vi "DynamicCursor.vi"() -> ()   [LabVIEW 2013]
doc: "This VI show how to create dynamic cursor."
uses:
  <vilib>/Utility/miscctls.llb/LVPointDoubleTypeDef.ctl
  <vilib>/Utility/miscctls.llb/LVCursorListTypeDef.ctl
panel:
  in  "Active Cursor":u32=3
  in  "Cursor.Cursor Position":T1
  out "XY Graph":cluster{"X":dbl, "Y":dbl}[](graph)
  # "1 Run this VI\n2 Change Cursor position\n3 Change Active Cursor"
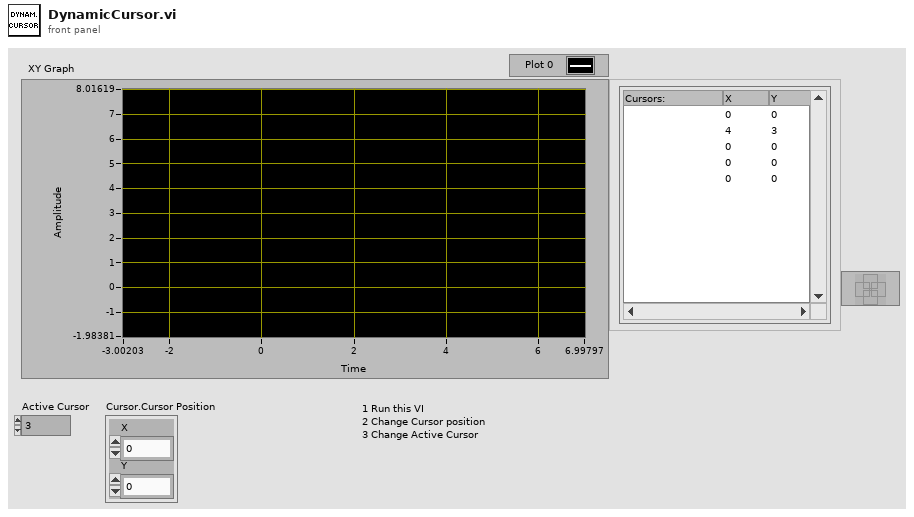
[diagram p1: front panel]
types:
  T1 = typedef "LVPointDoubleTypeDef.ctl" = cluster{"X":dbl, "Y":dbl}
  T2 = typedef "LVCursorListTypeDef.ctl" = cluster{"Name":string, "Color":u32, "Style":u8, "Point Style":u8, "Name Visible":bool, "Allow Drag":bool, "Cursor Mode":u32, "Plot":i32, "Index":i32, "Position":cluster{"X":dbl, "Y":dbl}, "X Scale":u32, "Y Scale":u32, "Watch Plots":i32[], "Watch All Plots":bool, "Plot Area":i32, "Label Offset":cluster{"X":dbl, "Y":dbl}}[]
  T3 = cluster{"Name":string, "Color":u32, "Style":u8, "Point Style":u8, "Name Visible":bool, "Allow Drag":bool, "Cursor Mode":u32, "Plot":i32, "Index":i32, "Position":cluster{"X":dbl, "Y":dbl}, "X Scale":u32, "Y Scale":u32, "Watch Plots":i32[], "Watch All Plots":bool, "Plot Area":i32, "Label Offset":cluster{"X":dbl, "Y":dbl}}
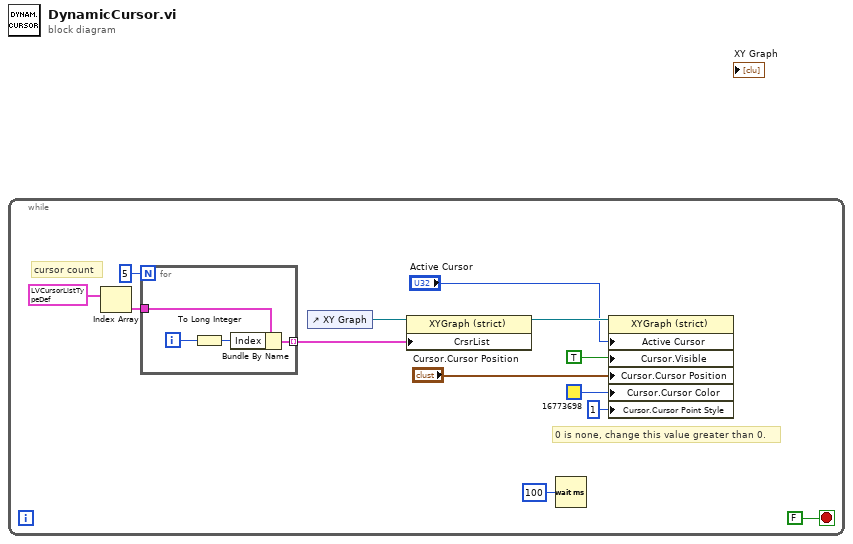
[diagram p0: block diagram]
diagram:
  n1 = while {
    stop <- FALSE stop-if-true
    # "cursor count"
    # "0 is none, change this value greater than 0."
    n2 = Index Array(array=T2 [{"Name"="", "Color"=0, "Style"=0, "Point Style"=0, "Name Visible"=FALSE, "Allow Drag"=FALSE, "Cursor Mode"=0, "Plot"=0, "Index"=0, "Position"={"X"=0.0, "Y"=0.0}, "X Scale"=0, "Y Scale"=0, "Watch Plots"=[], "Watch All Plots"=FALSE, "Plot Area"=0, "Label Offset"={"X"=0.0, "Y"=0.0}}] ("Cursor List")) -> (element=w7:T3)  [unwired: 1 in]
    n3 = for {
      N: 5 -> [_]
      tunnel: w7 -> [w17]
      tunnel: [w15] -> w6 mode=indexing
      i -> [w16]
      n4 = To Long Integer(number=w16) -> (32bit integer=w14:i32)
      n5 = Bundle By Name(cluster=w17, "Index"=w14) -> (w15:T3)
    }
    n6 = control-ref of="XY Graph"() -> (w11:refnum<vi>)
    n7 = property class="XYGraph (strict)"(reference=w11, "CrsrList"=w6) -> (reference out=w10:refnum<vi>)  [unwired: 1 in, 1 out]
    n8 = Wait (ms)(milliseconds to wait=u32 100) -> ()  [unwired: 1 out]
    n9 = property class="XYGraph (strict)"(reference=w10, "Active Cursor"="Active Cursor", "Cursor.Visible"=TRUE, "Cursor.Cursor Position"="Cursor.Cursor Position", "Cursor.Cursor Color"=u32 16773698, "Cursor.Cursor Point Style"=u8 1) -> ()  [unwired: 1 in, 2 out]
  }
